vi "DSF.Engine.Plugin.Rx.Async.vi"(8 "error in (no error)":errorcluster, 11 "Plugin in":refnum<class "DSF.Engine.Plugin.lvclass">) -> (0 "error out":errorcluster, 3 "Plugin out":refnum<class "DSF.Engine.Plugin.lvclass">)   [LabVIEW 2017, in "Data Sharing Framework Engine.lvlib" / "DSF.Engine.Plugin.lvclass"]
uses:
  DSF.Engine.Plugin.lvclass
  DSF.Engine.Plugin.lvclass/DSF.Engine.Plugin.ctl
  Timing/DSF.Engine.Timing.lvclass/DSF.Engine.Timing.ctl
  Transfer/DSF.Engine.Transfer Group.lvclass/DSF.Engine.Transfer Group.ctl
  Interface/DSF.Engine.Interface.Transceiver.Command.ctl
  Source/Data Sharing Framework Core/Engine/Debug/Debug Flags/Debug Flags.lvclass/Debug Flags.ctl
  Source/Data Sharing Framework Core/Engine/Debug/Debug Flags FIFO/Debug Flags FIFO.lvclass/Debug Flags FIFO.ctl
  Transfer/DSF.Engine.Transfer.lvclass/DSF.Engine.Transfer.ctl
  <vilib>/National Instruments/Memory Manager/Classes/Pointer/Memory.Pointer.lvclass/Memory.Pointer.ctl
  Timing/DSF.Engine.Timing.Is Active Cycle.vi
  Transfer/DSF.Engine.Transfer Group.Get Transfers.vi
  Transfer/DSF.Engine.Transfer.Get Inline Buffer.vi
  Transfer/DSF.Engine.Transfer.Get Intermediate Buffer.vi
  <vilib>/National Instruments/Memory Manager/Classes/Pointer/Memory.Pointer.Copy All.vi
  Transfer/DSF.Engine.Transfer Group.Return FIFO.Read.vi
  Timing/DSF.Engine.Timing.Iteration.Increment.vi
  Timing/DSF.Engine.Timing.Get Decimation.vi
  Timing/DSF.Engine.Timing.Get Offset.vi
  <vilib>/National Instruments/Memory Manager/Classes/Pointer/Memory.Pointer.Get Size.vi
  <vilib>/National Instruments/Memory Manager/Classes/Pointer/Memory.Pointer.Copy.vi
  Transfer/DSF.Engine.Transfer Group.Get Return FIFO.vi
  Transfer/DSF.Engine.Transfer Group.Get Debug Flags.vi
  Source/Data Sharing Framework Core/Engine/Debug/Debug Flags/Get FIFO Flags.vi
  Source/Data Sharing Framework Core/Engine/Debug/Debug Flags FIFO/Get Infinite Timeouts.vi
  <vilib>/National Instruments/Memory Manager/Classes/Pointer/Memory.Pointer.Copy.No Check.vi
  <vilib>/National Instruments/Memory Manager/Classes/Pointer/Memory.Pointer.Parameter Check.Subset.vi
  <vilib>/National Instruments/Memory Manager/Classes/Pointer/Memory.Pointer.Parameter Check.Null Pointer.vi
  <vilib>/National Instruments/Memory Manager/Classes/Pointer/Memory.Pointer.Get Address.vi
  <vilib>/National Instruments/Memory Manager/Classes/Pointer/Memory.Pointer.Errors.vi
  <vilib>/National Instruments/Memory Manager/Classes/Pointer/Memory.Pointer.Errors.Out of Bounds.vi
  <vilib>/National Instruments/Memory Manager/Classes/Pointer/Memory.Pointer.Errors.Null Pointer.vi
  <vilib>/NI/Static Error Handling/VIs/Static Error Handling.Source Buffer.Write.String.vi
  <vilib>/National Instruments/Memory Manager/Classes/Pointer/Memory.Pointer.Errors.Write Pointer Size.vi
  <vilib>/National Instruments/Memory Manager/Classes/Pointer/Memory.Pointer.Errors.Create Error.vi
  <vilib>/NI/Static Error Handling/VIs/Static Error Handling.Source Buffer.Write.Numeric.Scalar.Base10.vi
  <vilib>/NI/Static Error Handling/VIs/Static Error Handling.Source Buffer.Write.Numeric.Scalar.Base10 (U64).vi
  <vilib>/NI/Static Error Handling/VIs/Static Error Handling.Error Cluster Constant.vi
  <vilib>/NI/Static Error Handling/VIs/Static Error Handling.Error Cluster Constant (512B).vi
  <vilib>/NI/Static Error Handling/VIs/Static Error Handling.Parameters.Status.Set.vi
  <vilib>/NI/Static Error Handling/VIs/Static Error Handling.Parameters.Code.Set.vi
  <vilib>/NI/Static Error Handling/VIs/Static Error Handling.Parameters.VI Source.Set.vi
  <vilib>/National Instruments/Memory Manager/Constants/Memory.Constants.vi
  <vilib>/National Instruments/Memory Manager/Constants/Memory.Constants.Library Name.vi
  <vilib>/National Instruments/Memory Manager/Classes/Pointer/Memory.Pointer.Errors.Get Info.vi
  Pointer/DSF.Engine.Pointer.DBL.lvclass
  C:/Program Files (x86)/National Instruments/LabVIEW 2017/vi.lib/National Instruments/Memory Manager/Classes/Pointer/Memory.Pointer.lvclass
  Transfer/DSF.Engine.Transfer Group.Errors.vi
  Transfer/DSF.Engine.Transfer Group.Errors.Return Timeout.vi
  Transfer/DSF.Engine.Transfer Group.lvclass
  Timing/DSF.Engine.Timing.lvclass
  Interface/DSF.Engine.Interface.Transceiver.lvclass
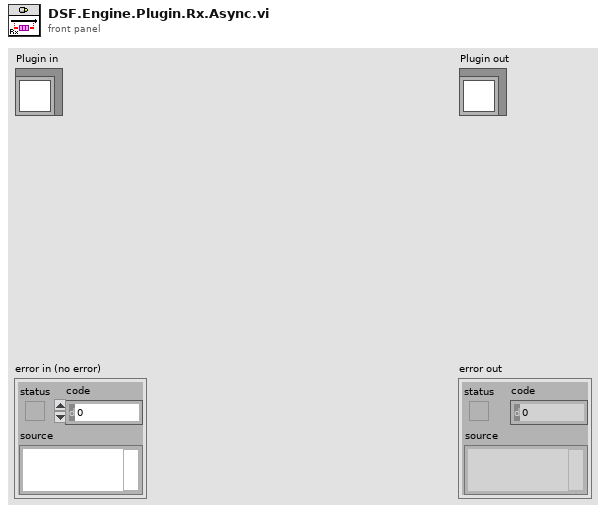
[diagram p1: front panel]
types:
  T1 = typedef "Data Sharing Framework Engine.lvlib/DSF.Engine.Interface.Transceiver.lvclass/DSF.Engine.Interface.Transceiver.Command.ctl" = enum8{"Set Base Pointer", "Rx", "Tx", "Shutdown"}
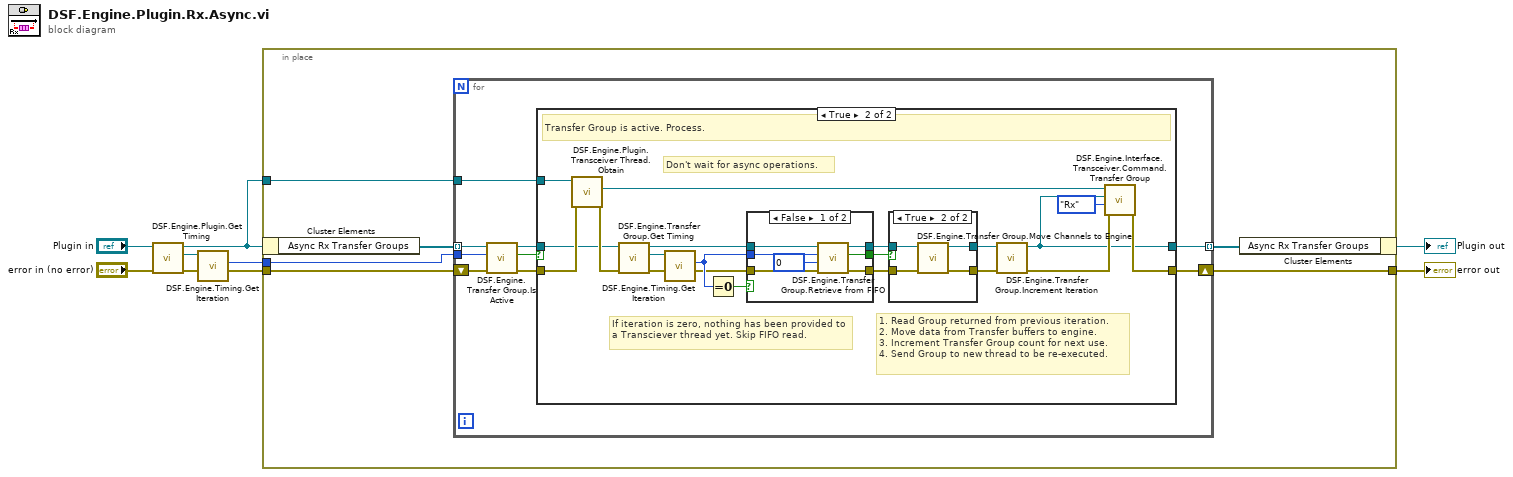
[diagram p0: block diagram]
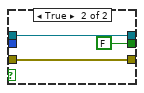
[diagram p3: hidden frame]
diagram:
  n1 = call "DSF.Engine.Plugin.Get Timing.vi"("Plugin in"="Plugin in") -> ("Timing"=w3:refnum<class "DSF.Engine.Timing.lvclass">, "Plugin out"=w4:refnum<class "DSF.Engine.Plugin.lvclass">)  [unwired: 9 in]
  n2 = call "DSF.Engine.Timing.Get Iteration.vi"("Timing in"=w3) -> ("Iteration"=w2:u64)  [unwired: 9 in, 1 out]
  n3 = in-place {
    in-place-border: "error in (no error)" -> [w13]
    in-place-border: [w12] -> w5
    in-place-border: w2 -> [w8]
    in-place-border: w4 -> [w9]
    n4 = in-place-cluster #1(w4) -> ("Async Rx Transfer Groups"=w11:refnum<class "DSF.Engine.Transfer Group.lvclass">[])
    n5 = for {
      tunnel: w11 -> [w21] mode=indexing
      tunnel: w8 -> [w20]
      shift-right: [w19] -> w12
      shift-left: w13 -> [w18]
      tunnel: [w15] -> w10 mode=indexing
      tunnel: w9 -> [w14]
      n6 = call "DSF.Engine.Transfer Group.Is Active.vi"("cycle count"=w20, "Transfer Group in"=w21) -> ("active this cycle?"=w17:bool, "Transfer Group out"=w16:refnum<class "DSF.Engine.Transfer Group.lvclass">)  [unwired: 8 in]
      n7 = case shown="True" w17 {
        tunnel: [w23 w29] -> w19
        tunnel: w18 -> [w23 w26]
        tunnel: w16 -> [w22 w24]
        tunnel: [w22 w28] -> w15
        tunnel: w14 -> [_ w35]
        frame False {
          # "Transfer Group is not active. Skip."
        }
        frame True {
          # "Don't wait for async operations."
          # "If iteration is zero, nothing has been provided to a Transciever thread yet. Skip FIFO read."
          # "1. Read Group returned from previous iteration.\n2. Move data from Transfer buffers to engine.\n3. Increment Transfer Group count for next use.\n4. Send Group to new thread to be re-executed."
          # "Transfer Group is active. Process."
          n8 = call "DSF.Engine.Plugin.Transceiver Thread.Obtain.vi"("error in (no error)"=w26, "Plugin in"=w35) -> ("error out"=w25:errorcluster, "Transceiver Thread"=w34:refnum<class "DSF.Engine.Interface.Transceiver.lvclass">)  [unwired: 7 in, 1 out]
          n9 = call "DSF.Engine.Transfer Group.Get Timing.vi"("Transfer Group in"=w24) -> ("Timing"=w40:refnum<class "DSF.Engine.Timing.lvclass">, "Transfer Group out"=w39:refnum<class "DSF.Engine.Transfer Group.lvclass">)  [unwired: 9 in]
          n10 = call "DSF.Engine.Timing.Get Iteration.vi"("Timing in"=w40) -> ("Iteration"=w31:u64)  [unwired: 9 in, 1 out]
          n11 = Equal To 0?(x=w31) -> (x = 0?=w41:bool)
          n12 = case shown="False" w41 {
            tunnel: w25 -> [w48 w51]
            tunnel: [w47 w49] -> w38
            tunnel: [w46 w51] -> w33
            tunnel: w39 -> [w45 w49]
            tunnel: w31 -> [w44 _]
            tunnel: [w43 FALSE ("iteration valid?")] -> w32
            frame False {
              n13 = call "DSF.Engine.Transfer Group.Retrieve from FIFO.vi"("error in (no error)"=w48, "timeout in ms (0)"=0, "expected iteration"=w44, "Transfer Group in"=w45) -> ("error out"=w46:errorcluster, "iteration valid?"=w43:bool, "Transfer Group out"=w47:refnum<class "DSF.Engine.Transfer Group.lvclass">)  [unwired: 5 in]
            }
            frame True {
            }
          }
          n14 = case shown="True" w32 {
            tunnel: w38 -> [w53 w54]
            tunnel: [w53 w55] -> w37
            tunnel: [w52 w56] -> w36
            tunnel: w33 -> [w52 w57]
            frame False {
            }
            frame True {
              n15 = call "DSF.Engine.Transfer Group.Move Channels to Engine.vi"("error in (no error)"=w57, "Transfer Group in"=w54) -> ("error out"=w56:errorcluster, "Transfer Group out"=w55:refnum<class "DSF.Engine.Transfer Group.lvclass">)  [unwired: 8 in]
            }
          }
          n16 = call "DSF.Engine.Transfer Group.Increment Iteration.vi"("error in (no error)"=w36, "Transfer Group in"=w37) -> ("error out"=w30:errorcluster, "Transfer Group out"=w28:refnum<class "DSF.Engine.Transfer Group.lvclass">)  [unwired: 8 in]
          n17 = call "DSF.Engine.Interface.Transceiver.Command.Transfer Group.vi"("error in (no error)"=w30, "Command"=DSF.Engine.Interface.Transceiver.Command."Rx", "Transfer Group"=w28, "Transceiver Interface in"=w34) -> ("error out"=w29:errorcluster)  [unwired: 6 in, 1 out]
        }
      }
    }
    n18 = in-place-cluster #1("Async Rx Transfer Groups"=w10) -> (→"Plugin out":refnum<class "DSF.Engine.Plugin.lvclass">)
  }
  "error out" <- w5
